vi "UpdatePOI.vi"(8 "error in (no error)":errorcluster, 10 "Points of Interest":T1[](array[typedef]) {"North" format="%#_10f"; "East" format="%#_8f"}, 11 "GenericMission in":refnum<class "GenericMission.lvclass">) -> (0 "error out":errorcluster, 3 "GenericMission out":refnum<class "GenericMission.lvclass">)   [LabVIEW 2013, in "GenericMission.lvclass"]
uses:
  GenericMission.lvclass
  Data/TypeDefs/UTM Location.ctl
  GenericMission.lvclass/GenericMission.ctl
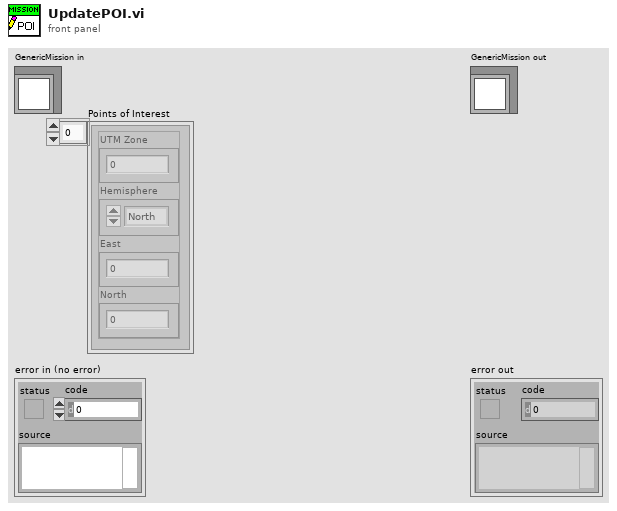
[diagram p1: front panel]
types:
  T1 = typedef "UTM Location.ctl" = cluster{"UTM Zone":dbl, "Hemisphere":enum16{"North", "South"}, "East":dbl, "North":dbl}
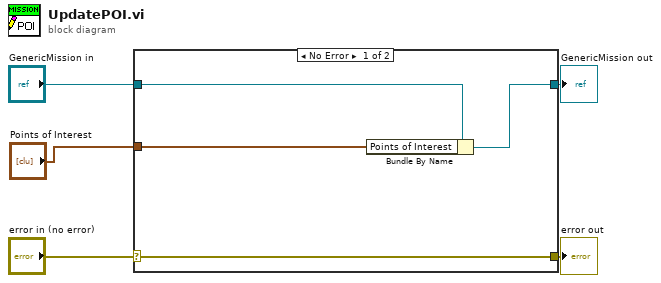
[diagram p0: block diagram]
diagram:
  n1 = case shown="No Error" "error in (no error)" {
    selector: "error in (no error)" -> [w9 w10]
    tunnel: [w9 w10] -> w4
    tunnel: [w8 w11] -> w2
    tunnel: "GenericMission in" -> [w7 w11]
    tunnel: "Points of Interest" -> [w6 _]
    frame No Error {
      n2 = Bundle By Name(cluster=w7, "Points of Interest"=w6) -> (w8:refnum<class "GenericMission.lvclass">)
    }
    frame Error {
    }
  }
  "error out" <- w4
  "GenericMission out" <- w2
